vi "P1_2_TiposDatos.vi"() -> ()   [LabVIEW 2020]
panel:
  out "Numeric":dbl
  out "salida palabra:":string
  in  "ingresa palabra:":string
  in  "encender led":bool
  out "salida numero":u8(slide) scale=0.0..100.0
  in  "Slide":dbl(slide) scale=0.0..10.0
  in  "Ingresa numero:":dbl
  out "led":bool
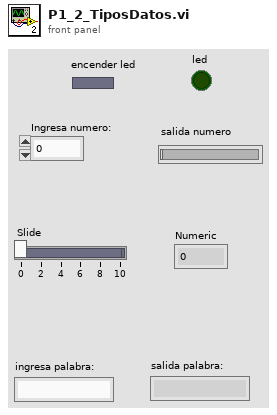
[diagram p1: front panel]
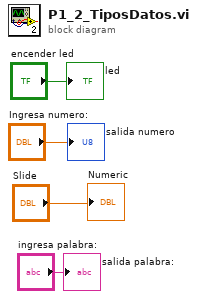
[diagram p0: block diagram]
diagram:
  "led" <- "encender led"
  "salida numero" <- "Ingresa numero:"
  "salida palabra:" <- "ingresa palabra:"
  "Numeric" <- "Slide"
